vi "Save bline to memory1.vi"(0 "PSOCTSpectral Bline":u16[](array[numeric]), 1 "action":T1=enum."Save(ThorOCT)", 5 "index (row)":i32, 9 "PSOCT Spatial Bline":sgl[](array[numeric]), 11 "error in":errorcluster) -> (15 "error out":errorcluster)   [LabVIEW 2018]
uses:
  Controls/Save Bline to Mem Control.ctl
  Controls/FGV Actions.ctl
  Controls/Queue Manager Actions.ctl
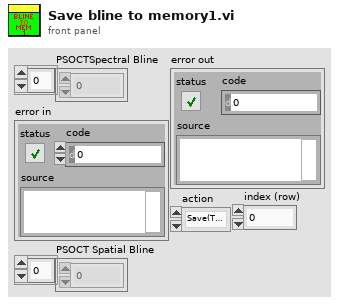
[diagram p1: front panel]
types:
  T1 = typedef "Save Bline to Mem Control.ctl" = enum16{"Output data", "Save(ThorOCT)", "Save(PSOCT)", "FFT and Save", "Uninit", "PSOCT Spectral buffer Set", "PSOCT Spatial buffer Set", "PSOCT Spectral buffer Init", "PSOCT Spatial buffer Init", "ThorOCT Spectral buffer Init", "ThorOCT Spatial buffer Init", "ThorOCT Spectral buffer Set", "ThorOCT Spatial buffer Set", "ThorOCT Spectral Save", "Alazar Spectral Save", "PSOCT save all", "Average"}
  T2 = typedef "FGV Actions.ctl" = enum16{"Init", "Set", "Get", "Clear"}
  T3 = typedef "System Parameters.ctl" = cluster{"Optical Parameters":T4, "Vibratome":T5, "Table Stages":T7, "Imaging Parameter":T10, "Galvo HW Parameters":cluster{"Analog Out Channel":tag, "Min Voltage":dbl, "Max Voltage":dbl, "Pixel Clock Source":tag, "Sample Rate":dbl, "Line Clock Out Ch":tag, "2P ready check":tag}, "Alazar parameters":T12, "Mosaic Paramter":cluster{"X Axis":cluster{"Start [mm]":dbl, "Steps [pts]":dbl, "End [mm]":dbl}, "Y Axis":cluster{"Start [mm]":dbl, "Steps [pts]":dbl, "End [mm]":dbl}, "Scan Pattern":enum16{"Uni-directional", "Bi-Directional", "Spiral Out", "Spiral In"}, "Overlap Options":cluster{"Overlap Type":enum16{"No Overlap", "X Only", "Y Only", "X and Y"}, "Percent Overlap":u8, "Justify":enum16{"Start", "Center", "End"}}}, "Manual Controls":T19, "Z stage setting":T23, "Attenuator":T24}
  T4 = typedef "Optical Parameters.ctl" = cluster{"Obj. Focal Length [mm]":dbl, "Scan Lens EFL[mm]":dbl, "Tube Lens EFL[mm]":dbl, "Galvo V Range (+/-)":dbl, "Galvo Max Half Angle [Deg]":dbl, "Max Galvo Range[%]":dbl}
  T5 = typedef "Vibratome Parameters.ctl" = cluster{"Pre Cut Dwell [s]":dbl, "Blade Frequency [RPM]":u16, "Slice Speed [mm/s]":dbl, "Post Cut Dwell [s]":dbl, "Ramp Time [s]":dbl, "Start X [mm]":dbl, "Start Y [mm]":dbl, "Slice Length [mm]":dbl, "Slice Axis":enum16{"X Axis", "Y Axis", "Z Axis"}, "Controller VISA Ref":refnum<visa-resource-name>, "Blade Frequency [Hz]":u16, "Analog Out Channel":tag, "Pixel Clock Source":tag, "Vib version":T6}
  T6 = typedef "vibratome.ctl" = enum16{"Vibratome1", "Vibratome3"}
  T7 = typedef "Translation Stage Parameters.ctl" = cluster{"X Stage":T8, "Y Stage":T8, "Z Stage":T8, "Attenuator":T8}
  T8 = typedef "Translation Stage Cluster.ctl" = cluster{"Position":dbl, "Is.Enabled?":bool, "Is.Connected?":bool, "Device SN":string, "AccelerationMaximum":dbl, "VelocityMaximum":dbl, "Acceleration":dbl, "Velocity":dbl, "waitTimeout (ms)":i32, "Model":T9, "Is.Homed?":bool, "MOVE":bool}
  T9 = typedef "Translation Stage Types.ctl" = enum16{"None", "Thorlabs LTS", "Thorlabs MLJ"}
  T10 = typedef "Imaging Parameters.ctl" = cluster{"Raster Scan Direction":T11, "Pixel Dwell Time [Clock Cycles]":u16, "Flyback Time [Clock Cycles]":u16, "XY Center [um]":cluster{"X":dbl, "Y":dbl}, "Pixel Step Size [um] X":dbl, "XY Image Size":enum16{"32 x 32", "64 x 64", "128 x 128", "256 x 256", "512 x 512", "1024 x 1024", "2048 x 2048"}, "Custom":bool, "Custom Size":cluster{"X":u16, "Y":u16}, "Line Averages":u16, "Pixel Step Size [um] Y":dbl}
  T11 = typedef "Scan Direction.ctl" = enum16{"Uni Directional", "Bi Directional", "None"}
  T12 = typedef "Alazar parameters.ctl" = cluster{"Trigger Settings":cluster{"General Trigger Settings":T13, "Trigger Engine 1":T14, "Trigger Engine 2":T14}, "Device ID":T15, "Ch A Input Control":T16, "Ch B Input Control":T16, "Acq Settings":T17, "Capture Clock":T18}
  T13 = typedef "General Trigger Settings.ctl" = cluster{"Trigger Operation":u32, "Coupling ID":u32, "Range ID":u32, "Delay":u32, "Timeout Ticks":u32, "Mode":u32, "Parameter":u32}
  T14 = typedef "Trigger Engine Controls.ctl" = cluster{"Trigger Engine":u32, "Source":u32, "Slope":u32, "Level":u32}
  T15 = typedef "Alazar Device ID.ctl" = cluster{"System ID":u32, "Board ID":u32}
  T16 = typedef "Channel Input Controls.ctl" = cluster{"Channel":u8, "Coupling":u32, "Range":u32, "Impedance":u32}
  T17 = typedef "Alazar Acquisition Settings.ctl" = cluster{"Record Length":u32, "Offset":u32, "Records Per Buffer":u32, "Records Count (Records/Acq)":u32, "Window Type":u32, "Footer":u32, "Samples per record":u32, "Output Format":u32}
  T18 = typedef "Clock Controls.ctl" = cluster{"Sample Rate":u32, "Decimation":u32, "Source":u32, "Edge":u32}
  T19 = typedef "Manual Controls.ctl" = cluster{"Data Path":path, "Save parameters":T20, "Acquisition mode":T21, "PSOCT Channel":u32, "Save data?":bool, "AIP rotation angle":dbl, "Pause acquisition?":bool, "Outgoing Mail Server (SMTP)":string, "Email":string, "Password":string, "Carrier 1":enum16{"T-Mobile", "AT&T", "Verizon", "Sprint"}, "phone number 1":string, "Subject":string, "Message":string, "Carrier 2":enum16{"T-Mobile", "AT&T", "Verizon", "Sprint"}, "phone number 2":string, "Check boundary?":bool, "Threshold":sgl, "Outputs for GPU FFT":T22}
  T20 = typedef "FFT parameters.ctl" = cluster{"start pixel":i32, "#pixels to save":i32}
  T21 = typedef "FFT mode.ctl" = enum16{"ThorOCT B line", "ThorOCT Spectral", "ThorOCT FFT", "Alazar B line", "Alazar FFT", "GPU FFT", "Alazar Spectral", "Simulation", "auto adjust focus", "Save all"}
  T22 = typedef "GPU FFT outputs.ctl" = enum16{"Amp + Phase diff", "Amp + Phase", "Amp only"}
  T23 = typedef "Vibratome Param.ctl" = cluster{"first cut height(mm)":dbl, "slice thickness[um]":dbl[], "#repetitions":u16, "image thickness(um)":dbl[], "#cycles per repetition":u16, "First image height(mm)":dbl, "Block?":bool[], "Z0":dbl, "fixed Z0?":bool}
  T24 = typedef "attenuator.ctl" = cluster{"Power after Objective (recalibrate every 6 month)":dbl[]}
  T25 = typedef "Queue Manager Actions.ctl" = enum16{"Init", "Enqueue", "Enqueue All", "Preview Queue", "Dequeue", "Get Status", "Flush Queue", "Flush All Queues", "Release All Queues", "Release Queue", "Enqueue at Opposite End"}
  T26 = typedef "Go Scan Actions.ctl" = enum16{"Init(ThorOCT Spatial)", "Init(ThorOCT Spectral)", "Init(GPU FFT)", "Init(Alazar FFT)", "Init Scan Head(ThorOCT Spectral)", "Init Scan Head(ThorOCT Spatial)", "Init Scan Head", "Init Table Stage", "Init Vibratome", "Generate Mosaic", "Generate Z Position", "Go to Image Z", "Go Image Home", "Go Mosaic", "Acquire Image(ThorOCT Spatial)", "Acquire Image(ThorOCT Spectral)", "Acquire Image(GPU FFT)", "Acquire Image(Alazar FFT)", "Go Vibratome", "Slice", "Finished(ThorOCT)", "Finished", "Init(Alazar Spectral)", "Go Vibratome3", "Tissue boundary"}
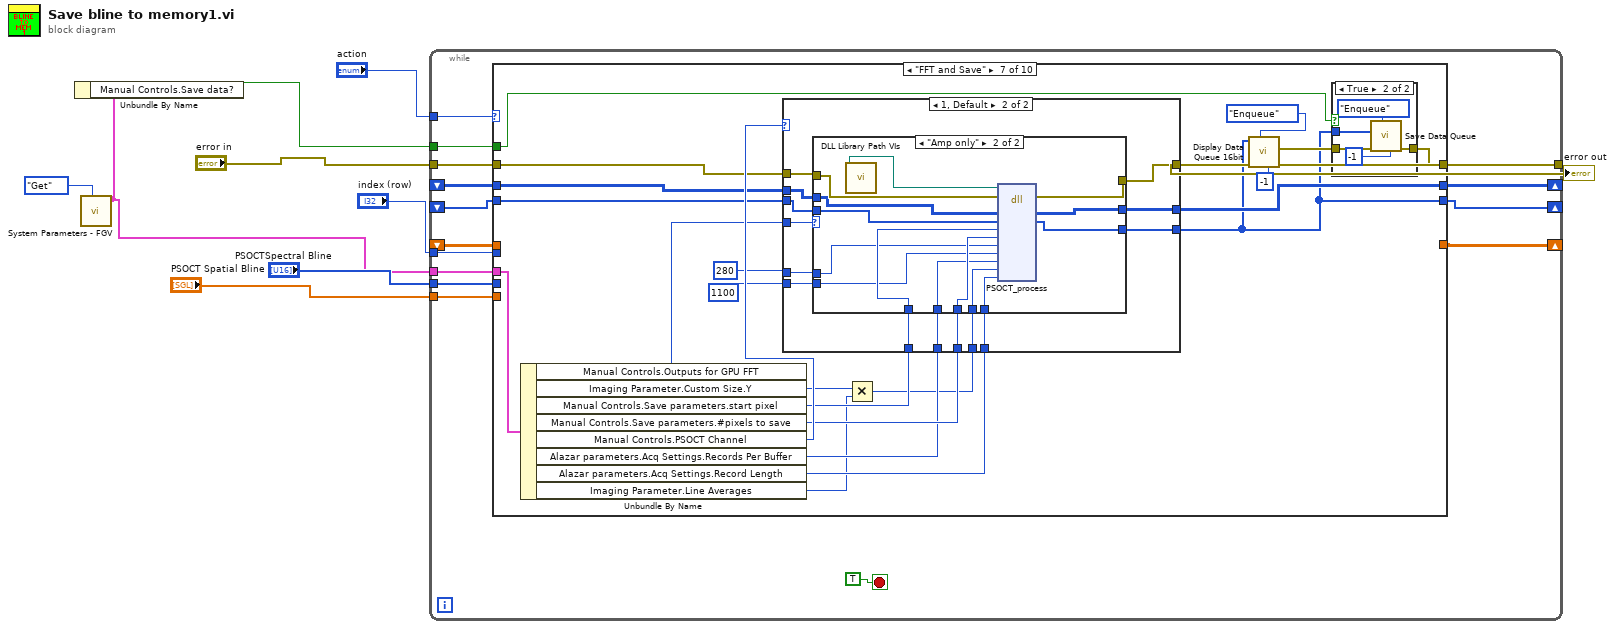
[diagram p0: block diagram]
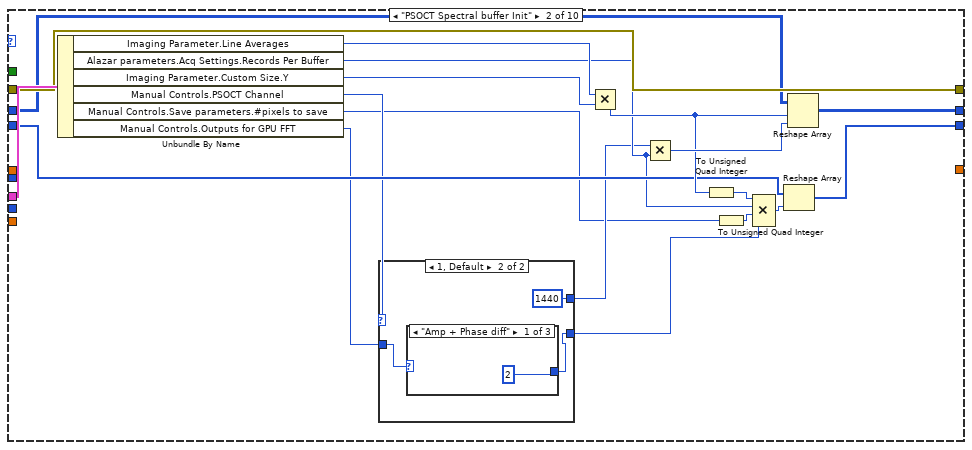
[diagram p3: hidden frame]
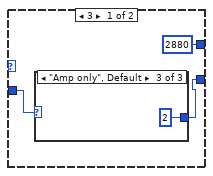
[diagram p4: hidden frame]
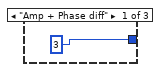
[diagram p5: hidden frame]
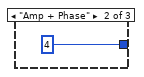
[diagram p6: hidden frame]
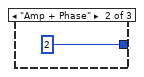
[diagram p7: hidden frame]
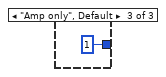
[diagram p8: hidden frame]
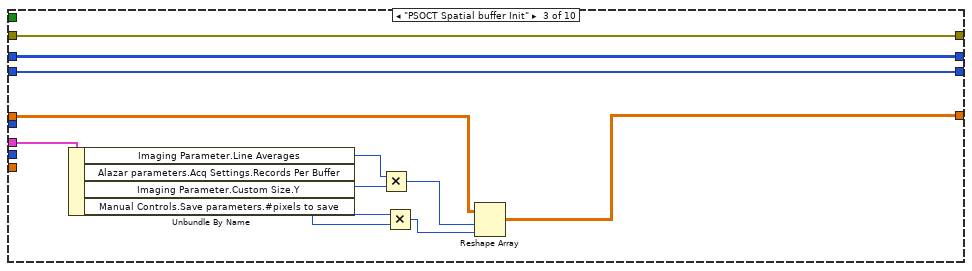
[diagram p9: hidden frame]
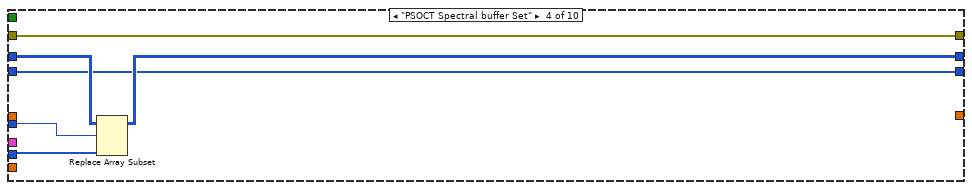
[diagram p10: hidden frame]
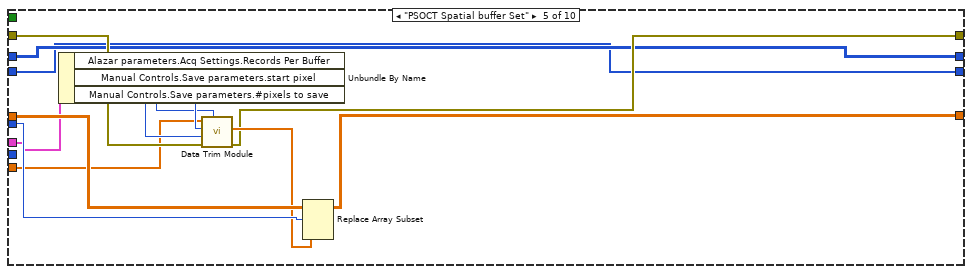
[diagram p11: hidden frame]
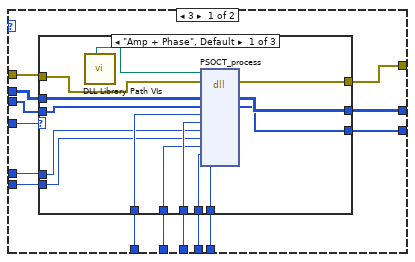
[diagram p13: hidden frame]
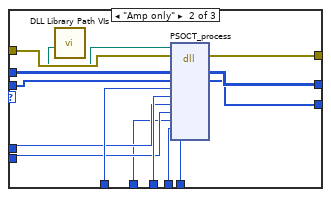
[diagram p14: hidden frame]
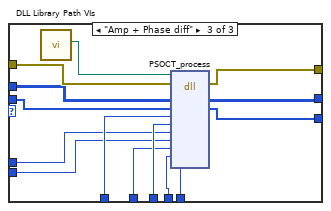
[diagram p15: hidden frame]
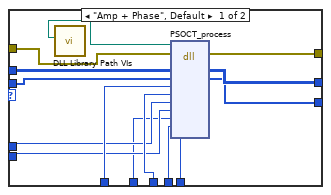
[diagram p16: hidden frame]
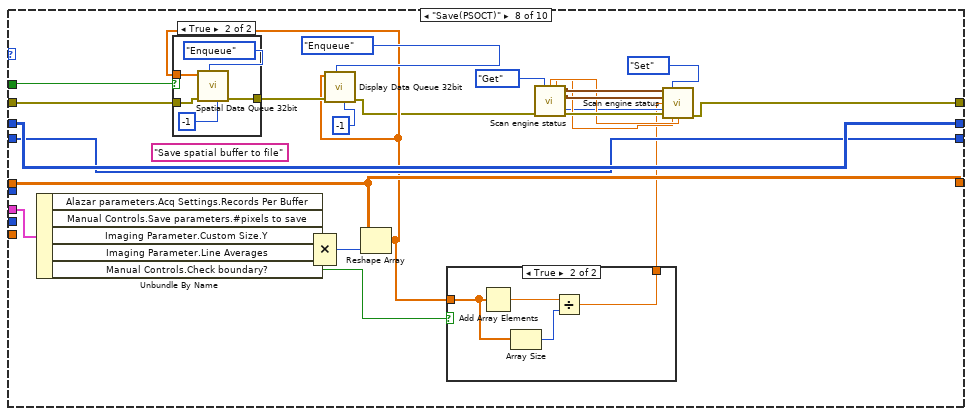
[diagram p18: hidden frame]
diagram:
  n1 = call "System Parameters - FGV.vi"("Actions"=FGV_Actions."Get") -> ("System Parameters [Out]"=w2:T3)  [unwired: 9 in, 1 out]
  n2 = Unbundle By Name(w2) -> ("Manual Controls.Save data?"=w1:bool)
  n3 = while {
    tunnel: "action" -> [w10]
    shift-right: [w22] -> _
    shift-left: _ -> [w17]
    tunnel: "PSOCTSpectral Bline" -> [w13]
    tunnel: "index (row)" -> [w11]
    tunnel: "error in" -> [w16]
    tunnel: w2 -> [w12]
    tunnel: [w23] -> w4
    shift-right: [w20] -> _
    shift-left: _ -> [w19]
    tunnel: "PSOCT Spatial Bline" -> [w14]
    tunnel: w1 -> [w15]
    shift-right: [w21] -> _
    shift-left: _ -> [w18]
    stop <- TRUE stop-if-true
    n4 = case shown="\"FFT and Save\"" w10 {
      tunnel: [w28 w46 w65 w74 w79 _ w100 w232 w261 w282] -> w22
      tunnel: w17 -> [w28 w37 w65 w77 w79 _ w109 w232 w261 w282]
      tunnel: w13 -> [_ _ _ w75 _ _ _ _ _ _]
      tunnel: w11 -> [_ _ _ w76 w88 _ _ _ _ _]
      tunnel: w16 -> [w26 w42 w66 w73 w84 w91 w110 w244 w264 w285]
      tunnel: w12 -> [_ w45 w71 _ w85 _ w113 w242 w279 _]
      tunnel: [w26 w42 w66 w73 w80 w91 w99 w219 w255 w284] -> w23
      tunnel: [w27 _ w63 _ w89 _ _ w243 w280 _] -> w20
      tunnel: w19 -> [w27 _ w62 _ w90 _ _ w243 w280 _]
      tunnel: w14 -> [_ _ _ _ w82 _ _ _ _ _]
      tunnel: w15 -> [_ _ _ _ _ _ w112 w234 _ _]
      tunnel: [w25 w41 w64 w72 w78 _ w95 w231 w260 w281] -> w21
      tunnel: w18 -> [w25 w36 w64 w72 w78 _ w108 w231 w260 w281]
      frame Default {
      }
      frame "PSOCT Spectral buffer Init" {
        n5 = Unbundle By Name(w45) -> ("Imaging Parameter.Line Averages"=w44:u16, "Alazar parameters.Acq Settings.Records Per Buffer"=w34:u32, "Imaging Parameter.Custom Size.Y"=w43:u16, "Manual Controls.PSOCT Channel"=w31:u32, "Manual Controls.Save parameters.#pixels to save"=w30:i32, "Manual Controls.Outputs for GPU FFT"=w29:T22)
        n6 = case shown="1, Default" w31 {
          tunnel: [w50 w56] -> w38
          tunnel: w29 -> [w49 w55]
          tunnel: [u32 2880 ("element") u32 1440 ("element")] -> w32
          frame 3 {
            n7 = case shown="\"Amp only\", Default" w49 {
              tunnel: [3 u64 4 ("element") u64 2 ("element")] -> w50
              frame "Amp + Phase diff" {
              }
              frame "Amp + Phase" {
              }
              frame "Amp only", Default {
              }
            }
          }
          frame 1, Default {
            n8 = case shown="\"Amp + Phase diff\"" w55 {
              tunnel: [2 u64 2 ("element") u64 1 ("element")] -> w56
              frame "Amp + Phase diff" {
              }
              frame "Amp + Phase" {
              }
              frame "Amp only", Default {
              }
            }
          }
        }
        n9 = Multiply(x=w44, y=w43) -> (x*y=w40:u16)
        n10 = Multiply(x=w32, y=w34) -> (x*y=w47:u32)
        n11 = To Unsigned Quad Integer(1:w40) -> (0:w35:u64)
        n12 = To Unsigned Quad Integer(1:w30) -> (0:w33:u64)
        n13 = Compound Arithmetic op=MULTIPLY(w35, w34, w33, w38) -> (w39:u64)
        n14 = Reshape Array(w36, w39) -> (w41:u16[])
        n15 = Reshape Array(w37, w40, w47) -> (w46:u16[][])
      }
      frame "PSOCT Spatial buffer Init" {
        n16 = Unbundle By Name(w71) -> ("Imaging Parameter.Line Averages"=w68:u16, "Alazar parameters.Acq Settings.Records Per Buffer"=w69:u32, "Imaging Parameter.Custom Size.Y"=w67:u16, "Manual Controls.Save parameters.#pixels to save"=w70:i32)
        n17 = Multiply(x=w68, y=w67) -> (x*y=w61:u16)
        n18 = Multiply(x=w69, y=w70) -> (x*y=w60:u32)
        n19 = Reshape Array(w62, w61, w60) -> (w63:sgl[][])
      }
      frame "PSOCT Spectral buffer Set" {
        n20 = Replace Array Subset(array=w77, new element=w75, index (row)=w76) -> (w74:u16[][])  [unwired: 1 in]
      }
      frame "PSOCT Spatial buffer Set" {
        n21 = Unbundle By Name(w85) -> ("Alazar parameters.Acq Settings.Records Per Buffer"=w87:u32, "Manual Controls.Save parameters.start pixel"=w86:i32, "Manual Controls.Save parameters.#pixels to save"=w81:i32)
        n22 = call "Data Trim Module.vi"("#pixels to save"=w81, "error in"=w84, "start pixel"=w86, "#A-lines"=w87, "1D Array in"=w82) -> ("error out"=w80:errorcluster, "array for saving"=w83:sgl[])  [unwired: 5 in]
        n23 = Replace Array Subset(array=w90, new element=w83, index (row)=w88) -> (w89:sgl[][])  [unwired: 1 in]
      }
      frame "Uninit" {
      }
      frame "FFT and Save" {
        n24 = Unbundle By Name(w113) -> ("Manual Controls.Outputs for GPU FFT"=w101:T22, "Imaging Parameter.Custom Size.Y"=w94:u16, "Manual Controls.Save parameters.start pixel"=w107:i32, "Manual Controls.Save parameters.#pixels to save"=w106:i32, "Manual Controls.PSOCT Channel"=w111:u32, "Alazar parameters.Acq Settings.Records Per Buffer"=w103:u32, "Alazar parameters.Acq Settings.Record Length"=w102:u32, "Imaging Parameter.Line Averages"=w93:u16)
        n25 = Multiply(x=w94, y=w93) -> (x*y=w92:u16)
        n26 = case shown="1, Default" w111 {
          tunnel: w110 -> [w127 w183]
          tunnel: w109 -> [w126 w182]
          tunnel: w108 -> [w125 w181]
          tunnel: w107 -> [w124 w180]
          tunnel: w106 -> [w123 w179]
          tunnel: i16 280 ("a") -> [w122 w178]
          tunnel: i16 1100 ("b") -> [w121 w177]
          tunnel: w103 -> [w120 w176]
          tunnel: w92 -> [w119 w175]
          tunnel: w102 -> [w118 w174]
          tunnel: [w115 w171] -> w97
          tunnel: [w114 w170] -> w100
          tunnel: [w117 w173] -> w95
          tunnel: w101 -> [w116 w172]
          frame 3 {
            n27 = case shown="\"Amp + Phase\", Default" w116 {
              tunnel: w127 -> [w141 w155 w169]
              tunnel: w126 -> [w138 w152 w168]
              tunnel: w125 -> [w137 w151 w167]
              tunnel: w124 -> [w136 w150 w166]
              tunnel: w123 -> [w135 w149 w165]
              tunnel: w122 -> [w134 w148 w164]
              tunnel: w121 -> [w133 w147 w163]
              tunnel: w120 -> [w132 w146 w162]
              tunnel: w119 -> [w131 w145 w161]
              tunnel: w118 -> [w130 w144 w160]
              tunnel: [w129 w143 w159] -> w115
              tunnel: [w140 w154 w158] -> w114
              tunnel: [w139 w153 w157] -> w117
              frame "Amp + Phase", Default {
                n28 = call "DLL Library Path VIs.vi"() -> ("GPU FFT amp amp phase phase"=w128:path)  [unwired: 5 in, 6 out]
                n29 = dll-call lib="C:/Project/SerialSectionOCT/SerialSectOCT/Labview Software/DLL/CUDA_FFT_2_channel_amp_amp_phase_phase.dll" fn="PSOCT_process"(path in=w128, error in=w141, "h_signal"=w138, "h_processed_signal"=w137, "Z0"=w136, "DEPTH"=w135, "a"=w134, "b"=w133, "NALINES"=w132, "NBLINES"=w131, "SAMPLES"=w130) -> (error out=w129:errorcluster, "h_signal"=w140:u16[][], "h_processed_signal"=w139:u16[])  [unwired: 9 in, 1 out]
              }
              frame "Amp only" {
                n30 = call "DLL Library Path VIs.vi"() -> ("GPU FFT amp amp"=w142:path)  [unwired: 5 in, 6 out]
                n31 = dll-call lib="C:/Project/SerialSectionOCT/SerialSectOCT/Labview Software/DLL/CUDA_FFT_2_channel_amp_amp.dll" fn="PSOCT_process"(path in=w142, error in=w155, "h_signal"=w152, "h_processed_signal"=w151, "Z0"=w150, "DEPTH"=w149, "a"=w148, "b"=w147, "NALINES"=w146, "NBLINES"=w145, "SAMPLES"=w144) -> (error out=w143:errorcluster, "h_signal"=w154:u16[][], "h_processed_signal"=w153:u16[])  [unwired: 9 in, 1 out]
              }
              frame "Amp + Phase diff" {
                n32 = call "DLL Library Path VIs.vi"() -> ("GPU FFT amp amp phase diff"=w156:path)  [unwired: 5 in, 6 out]
                n33 = dll-call lib="C:/Project/SerialSectionOCT/SerialSectOCT/Labview Software/DLL/CUDA_FFT_2_channel_amp_amp_phasediff.dll" fn="PSOCT_process"(path in=w156, error in=w169, "h_signal"=w168, "h_processed_signal"=w167, "Z0"=w166, "DEPTH"=w165, "a"=w164, "b"=w163, "NALINES"=w162, "NBLINES"=w161, "SAMPLES"=w160) -> (error out=w159:errorcluster, "h_signal"=w158:u16[][], "h_processed_signal"=w157:u16[])  [unwired: 9 in, 1 out]
              }
            }
          }
          frame 1, Default {
            n34 = case shown="\"Amp only\"" w172 {
              tunnel: w183 -> [w197 w211]
              tunnel: w182 -> [w194 w210]
              tunnel: w181 -> [w193 w209]
              tunnel: w180 -> [w192 w208]
              tunnel: w179 -> [w191 w207]
              tunnel: w178 -> [w190 w206]
              tunnel: w177 -> [w189 w205]
              tunnel: w176 -> [w188 w204]
              tunnel: w175 -> [w187 w203]
              tunnel: w174 -> [w186 w202]
              tunnel: [w185 w201] -> w171
              tunnel: [w196 w200] -> w170
              tunnel: [w195 w199] -> w173
              frame "Amp + Phase", Default {
                n35 = call "DLL Library Path VIs.vi"() -> ("GPU FFT single amp phase"=w184:path)  [unwired: 5 in, 6 out]
                n36 = dll-call lib="C:/Project/SerialSectionOCT/SerialSectOCT/Labview Software/DLL/CUDA_FFT_1_channel_amp_phase.dll" fn="PSOCT_process"(path in=w184, error in=w197, "h_signal"=w194, "h_processed_signal"=w193, "Z0"=w192, "DEPTH"=w191, "a"=w190, "b"=w189, "NALINES"=w188, "NBLINES"=w187, "SAMPLES"=w186) -> (error out=w185:errorcluster, "h_signal"=w196:u16[][], "h_processed_signal"=w195:u16[])  [unwired: 9 in, 1 out]
              }
              frame "Amp only" {
                n37 = call "DLL Library Path VIs.vi"() -> ("GPU FFT single amp"=w198:path)  [unwired: 5 in, 6 out]
                n38 = dll-call lib="C:/Project/SerialSectionOCT/SerialSectOCT/Labview Software/DLL/CUDA_FFT_1_channel_amp.dll" fn="PSOCT_process"(path in=w198, error in=w211, "h_signal"=w210, "h_processed_amps"=w209, "Z0"=w208, "DEPTH"=w207, "a"=w206, "b"=w205, "NALINES"=w204, "NBLINES"=w203, "SAMPLES"=w202) -> (error out=w201:errorcluster, "h_signal"=w200:u16[][], "h_processed_amps"=w199:u16[])  [unwired: 9 in, 1 out]
              }
            }
          }
        }
        n39 = call "Display Data Queue 16bit.vi"("timeout in ms (-1)"=-1, "Action"=Queue_Manager_Actions."Enqueue", "data in"=w95) -> ()  [unwired: 5 in, 4 out]
        n40 = case shown="True" w112 {
          tunnel: w97 -> [w212 w217]
          tunnel: [w212 w216] -> w99
          tunnel: w95 -> [_ w213]
          frame False {
          }
          frame True {
            n41 = call "Save Data Queue.vi"("timeout in ms (-1)"=-1, "Action"=Queue_Manager_Actions."Enqueue", "error in (no error)"=w217, "data in"=w213) -> ("error out"=w216:errorcluster)  [unwired: 4 in, 3 out]
          }
        }
      }
      frame "Save(PSOCT)" {
        (unwired) "Save spatial buffer to file"
        n42 = Unbundle By Name(w242) -> ("Alazar parameters.Acq Settings.Records Per Buffer"=w241:u32, "Manual Controls.Save parameters.#pixels to save"=w240:i32, "Imaging Parameter.Custom Size.Y"=w239:u16, "Imaging Parameter.Line Averages"=w233:u16, "Manual Controls.Check boundary?"=w230:bool)
        n43 = Compound Arithmetic op=MULTIPLY(w241, w240, w239, w233) -> (w238:u32)
        n44 = Reshape Array(w243, w238) -> (w229:sgl[])
        n45 = case shown="True" w234 {
          tunnel: w244 -> [w249 w254]
          tunnel: [w249 w253] -> w237
          tunnel: w229 -> [_ w250]
          frame False {
          }
          frame True {
            n46 = call "Spatial Data Queue 32bit.vi"("timeout in ms (-1)"=-1, "Action"=Queue_Manager_Actions."Enqueue", "error in (no error)"=w254, "data in"=w250) -> ("error out"=w253:errorcluster)  [unwired: 4 in, 3 out]
          }
        }
        n47 = call "Display Data Queue 32bit.vi"("timeout in ms (-1)"=-1, "Action"=Queue_Manager_Actions."Enqueue", "error in (no error)"=w237, "data in"=w229) -> ("error out"=w220:errorcluster)  [unwired: 4 in, 3 out]
        n48 = case shown="True" w230 {
          tunnel: w229 -> [_ w245]
          tunnel: [_ w246] -> w218
          frame False {
          }
          frame True {
            n49 = Add Array Elements(numeric array=w245) -> (sum=w248:sgl)
            n50 = Array Size(array=w245) -> (size(s)=w247:i32)
            n51 = Divide(x=w248, y=w247) -> (x/y=w246:sgl)
          }
        }
        n52 = call "Scan engine status.vi"("Actions"=FGV_Actions."Get", "Error In"=w220) -> ("slice plane out"=w223:dbl, "image plane out"=w222:dbl, "XY Graph out"=w225:cluster{"X":dbl, "Y":dbl}[], "Current Position out"=w226:cluster{"X":dbl, "Y":dbl}, "Current state out"=w221:T26, "Error Out"=w227:errorcluster)  [unwired: 7 in, 1 out]
        n53 = call "Scan engine status.vi"("XY Graph in"=w225, "Actions"=FGV_Actions."Set", "Current Position in"=w226, "average"=w218, "Current state in"=w221, "Error In"=w227, "image plane"=w222, "slice plane"=w223) -> ("Error Out"=w219:errorcluster)  [unwired: 1 in, 6 out]
      }
      frame "Average" {
        (unwired) "Calculate average pixel value"
        n54 = Unbundle By Name(w279) -> ("Alazar parameters.Acq Settings.Records Per Buffer"=w278:u32, "Manual Controls.Save parameters.#pixels to save"=w277:i32, "Imaging Parameter.Custom Size.Y"=w276:u16, "Imaging Parameter.Line Averages"=w274:u16)
        n55 = Compound Arithmetic op=MULTIPLY(w278, w277, w276, w274) -> (w275:u32)
        n56 = call "Scan engine status.vi"("Actions"=FGV_Actions."Get", "Error In"=w264) -> ("slice plane out"=w266:dbl, "image plane out"=w265:dbl, "XY Graph out"=w268:cluster{"X":dbl, "Y":dbl}[], "Current Position out"=w269:cluster{"X":dbl, "Y":dbl}, "Current state out"=w262:T26, "Error Out"=w270:errorcluster)  [unwired: 7 in, 1 out]
        n57 = Reshape Array(w280, w275) -> (w256:sgl[])
        n58 = Add Array Elements(numeric array=w256) -> (sum=w273:sgl)
        n59 = Array Size(array=w256) -> (size(s)=w272:i32)
        n60 = Divide(x=w273, y=w272) -> (x/y=w263:sgl)
        n61 = call "Scan engine status.vi"("XY Graph in"=w268, "Actions"=FGV_Actions."Set", "Current Position in"=w269, "average"=w263, "Current state in"=w262, "Error In"=w270, "image plane"=w265, "slice plane"=w266) -> ("Error Out"=w257:errorcluster)  [unwired: 1 in, 6 out]
        n62 = call "Display Data Queue 32bit.vi"("timeout in ms (-1)"=-1, "Action"=Queue_Manager_Actions."Enqueue", "error in (no error)"=w257, "data in"=w256) -> ("error out"=w255:errorcluster)  [unwired: 4 in, 3 out]
      }
      frame "Alazar Spectral Save" {
        n63 = call "Spectral Save Queue.vi"("timeout in ms (-1)"=-1, "Action"=Queue_Manager_Actions."Enqueue", "error in (no error)"=w285, "data in"=w282) -> ("error out"=w284:errorcluster)  [unwired: 4 in, 3 out]
      }
    }
  }
  "error out" <- w4
